vi "verify exit message.vi"(8 "error in (no error)":errorcluster, 10 "message":string, 11 "Socket in":refnum<class "Socket.lvclass">) -> (0 "error out":errorcluster, 3 "Socket out":refnum<class "Socket.lvclass">)   [LabVIEW 2018, in "Socket.lvclass"]
uses:
  Socket.lvclass
  Socket.lvclass/Socket.ctl
  State Machine/CM_State Machine.lvclass
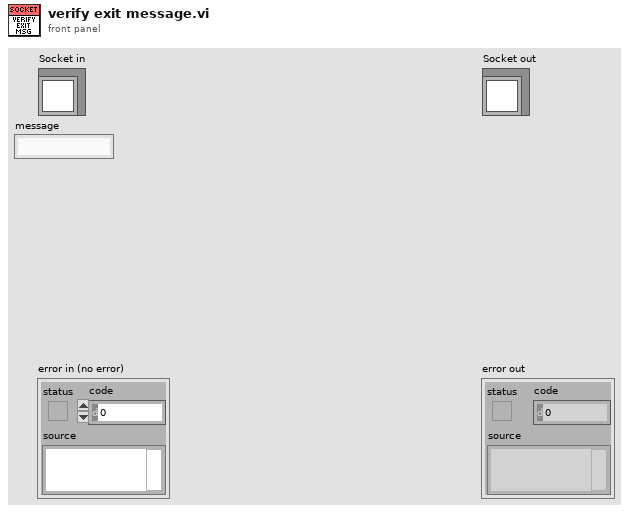
[diagram p1: front panel]
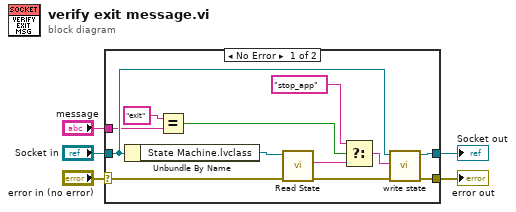
[diagram p0: block diagram]
diagram:
  n1 = case shown="No Error" "error in (no error)" {
    selector: "error in (no error)" -> [w10 w19]
    tunnel: [w12 w19] -> w4
    tunnel: [w13 w18] -> w2
    tunnel: "Socket in" -> [w14 w18]
    tunnel: "message" -> [w6 _]
    frame No Error {
      n2 = Unbundle By Name(w14) -> ("State Machine.lvclass"=w7:refnum<class "CM_State Machine.lvclass">)
      n3 = Equal?(x="exit" ("new state"), y=w6) -> (x = y?=w16:bool)
      n4 = call-dynamic "Read State.vi"("error in (no error)"=w10, "State Machine in"=w7) -> ("error out"=w9:errorcluster, "State"=w8:string)  [unwired: 7 in, 1 out]
      n5 = Select(t="stop_app", s=w16, f=w8) -> (s? t:f=w17:string)
      n6 = call "write state.vi"("error in (no error)"=w9, "State"=w17, "Socket in"=w14) -> ("error out"=w12:errorcluster, "Socket out"=w13:refnum<class "Socket.lvclass">)  [unwired: 7 in]
    }
    frame Error {
    }
  }
  "error out" <- w4
  "Socket out" <- w2
